vi "Test.vi"() -> ()   [LabVIEW 2021]
panel:
  out "error out":errorcluster
  out "file or folder exists?":bool
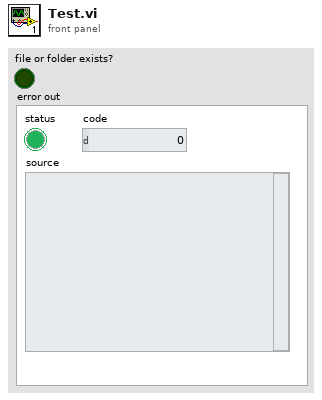
[diagram p1: front panel]
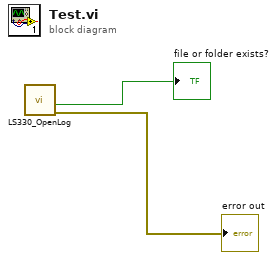
[diagram p0: block diagram]
diagram:
  n1 = call "LS330_OpenLog.vi"() -> ("error out"=→"error out":errorcluster, "file or folder exists?"=→"file or folder exists?":bool)  [unwired: 9 in, 1 out]
